vi "Clear Methods Registration.vi"(8 "error in (no error)":errorcluster, 11 "Server class in":refnum<vi>) -> (0 "error out":errorcluster, 3 "Server class out":refnum<vi>)   [LabVIEW 2019, in "gRPC Scripting Tools.lvlib"]
uses:
  gRPC Scripting Tools.lvlib
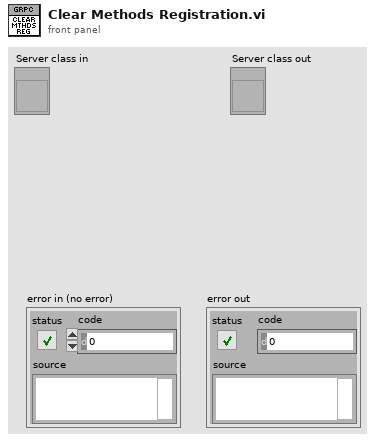
[diagram p1: front panel]
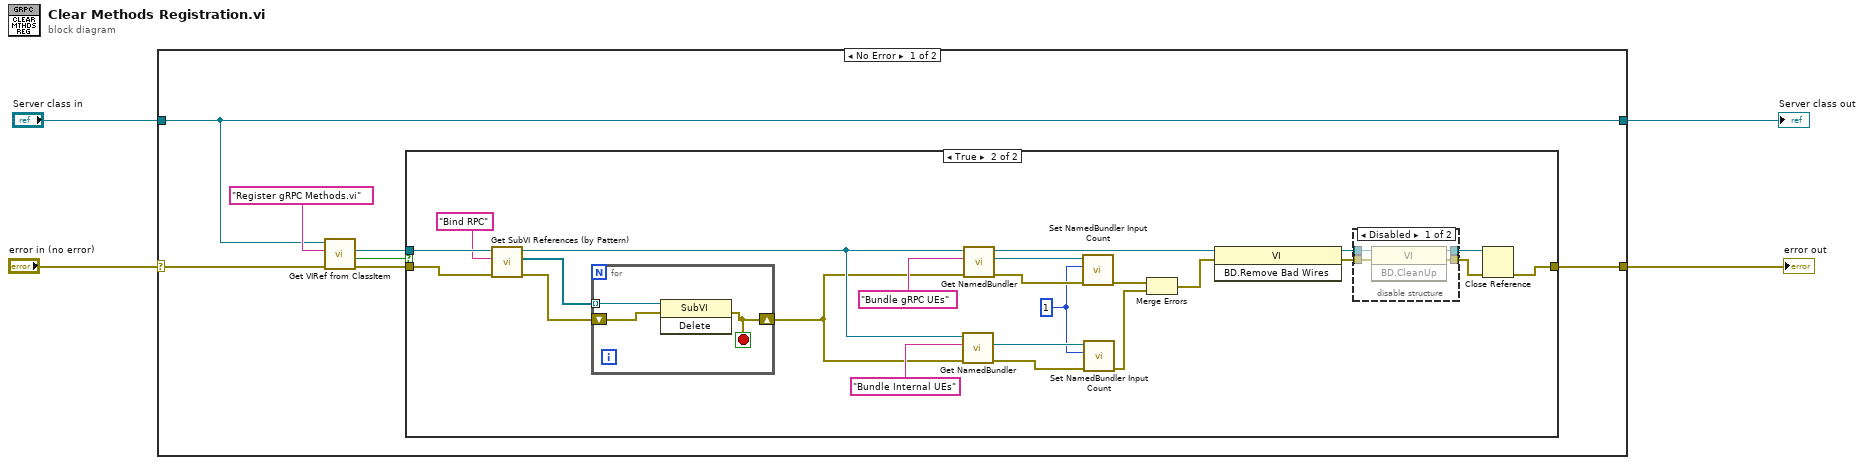
[diagram p0: block diagram]
diagram:
  n1 = case shown="No Error" "error in (no error)" {
    selector: "error in (no error)" -> [w10 w45]
    tunnel: [w6 w45] -> w4
    tunnel: "Server class in" -> [w9 w46]
    tunnel: [w9 w46] -> w1
    frame No Error {
      n2 = call "Get VIRef from ClassItem.vi"("error in (no error)"=w10, "Item Name"="Register gRPC Methods.vi", "LVClassLibrary in"=w9) -> ("error out"=w8:errorcluster, "Found ?"=w5:bool, "VIref out"=w7:refnum<vi>)  [unwired: 5 in, 1 out]
      n3 = case shown="True" w5 {
        tunnel: w8 -> [w12 w35]
        tunnel: w7 -> [_ w34]
        tunnel: [w12 w26] -> w6
        frame False {
        }
        frame True {
          w16 = 1 ("Numeric")
          n4 = call "Get SubVI References (by Pattern).vi"("error in (no error)"=w35, "SubVI Name Pattern"="Bind RPC" ("regular expression"), "VI ref in"=w34) -> ("error out"=w32:errorcluster, "SubVI refs"=w31:refnum<vi>[], "VI ref out"=w19:refnum<vi>)  [unwired: 6 in]
          n5 = for {
            tunnel: w31 -> [w44] mode=indexing
            shift-right: [w42] -> w17
            shift-left: w32 -> [w43]
            stop <- w42 stop-if-true
            n6 = invoke class="SubVI" method="Delete"(reference=w44, error in=w43) -> (error out=w42:errorcluster)  [unwired: 1 in, 2 out]
          }
          n7 = call "Get NamedBundler.vi"("error in (no error)"=w17, "Label"="Bundle Internal UEs" ("name/order"), "Owner VI in"=w19) -> ("error out"=w21:errorcluster, "NamedBundler ref out"=w22:refnum<vi>)  [unwired: 5 in, 2 out]
          n8 = call "Get NamedBundler.vi"("error in (no error)"=w17, "Label"="Bundle gRPC UEs" ("name/order"), "Owner VI in"=w19) -> ("error out"=w23:errorcluster, "NamedBundler ref out"=w25:refnum<vi>, "Owner VI out"=w20:refnum<vi>)  [unwired: 5 in, 1 out]
          n9 = call "Set NamedBundler Input Count.vi"("error in (no error)"=w23, "Numeric"=w16, "NamedBundler in"=w25) -> ("error out"=w15:errorcluster)  [unwired: 7 in, 1 out]
          n10 = call "Set NamedBundler Input Count.vi"("error in (no error)"=w21, "Numeric"=w16, "NamedBundler in"=w22) -> ("error out"=w14:errorcluster)  [unwired: 7 in, 1 out]
          n11 = Merge Errors(w15, w14) -> (w13:errorcluster)
          n12 = invoke class="VI" method="BD.Remove Bad Wires"(reference=w20, error in=w13) -> (reference out=w30:refnum<vi>, error out=w29:errorcluster)  [unwired: 1 in, 1 out]
          n13 = disable-structure shown="Disabled" {
            disable-tunnel: w30 -> [w39 w40]
            disable-tunnel: w29 -> [w38 w41]
            disable-tunnel: [w37 w41] -> w28
            disable-tunnel: [w36 w40] -> w27
            frame Disabled {
              n14 = invoke class="VI" method="BD.CleanUp"(reference=w39, error in=w38) -> (reference out=w36:refnum<vi>, error out=w37:errorcluster)  [unwired: 1 in, 1 out]
            }
            frame Enabled {
            }
          }
          n15 = Close Reference(reference=w27, error in (no error)=w28) -> (error out=w26:errorcluster)
        }
      }
    }
    frame Error {
    }
  }
  "error out" <- w4
  "Server class out" <- w1
